vi "PulseParseCamera.vi"(0 "Pars String":string) -> (1 "aux camera pars":T1, 2 "main camera pars":T2)   [LabVIEW 2017]
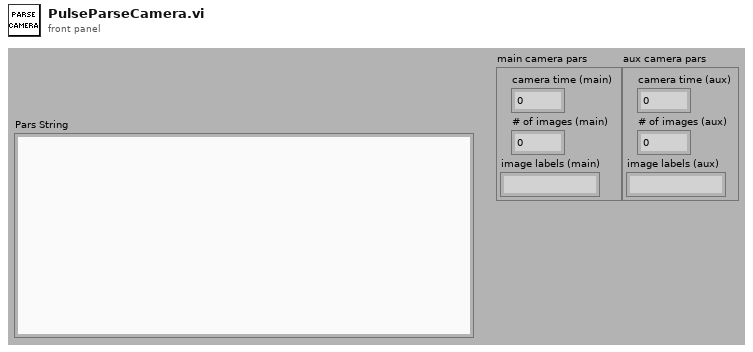
[diagram p1: front panel]
types:
  T1 = cluster{"camera time (aux)":i32, "# of images (aux)":i32, "image labels (aux)":string}
  T2 = cluster{"camera time (main)":i32, "# of images (main)":i32, "image labels (main)":string}
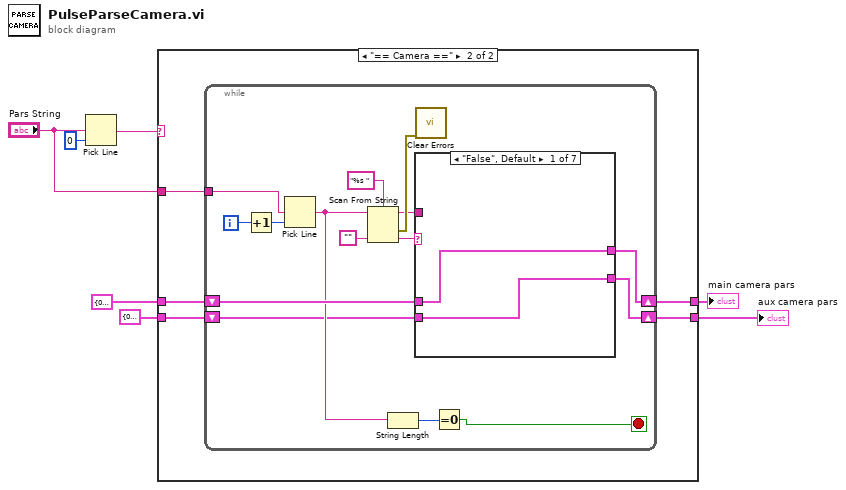
[diagram p0: block diagram]
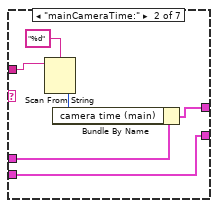
[diagram p3: hidden frame]
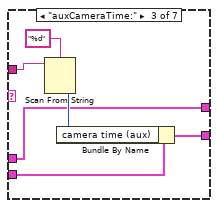
[diagram p4: hidden frame]
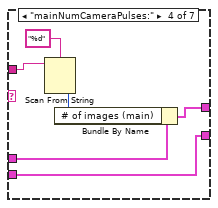
[diagram p5: hidden frame]
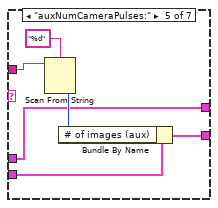
[diagram p6: hidden frame]
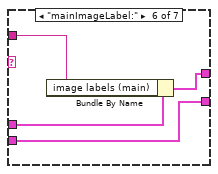
[diagram p7: hidden frame]
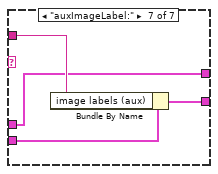
[diagram p8: hidden frame]
diagram:
  n1 = Pick Line(multi-line string="Pars String", line index=0) -> (output string=w6:string)  [unwired: 1 in]
  n2 = case shown="\"== Camera ==\"" w6 {
    tunnel: T2 {"camera time (main)"=0, "# of images (main)"=0, "image labels (main)"=""} ("Pars cluster 2") -> [w9 w14]
    tunnel: [w9 w13] -> w2
    tunnel: "Pars String" -> [_ w12]
    tunnel: T1 {"camera time (aux)"=0, "# of images (aux)"=0, "image labels (aux)"=""} ("Pars cluster 2") -> [w8 w11]
    tunnel: [w8 w10] -> w1
    frame "False", Default {
    }
    frame "== Camera ==" {
      n3 = while {
        shift-right: [w23] -> w13
        shift-left: w14 -> [w24]
        tunnel: w12 -> [w22]
        shift-right: [w15] -> w10
        shift-left: w11 -> [w16]
        i -> [w28]
        stop <- w19 stop-if-true
        n4 = Increment(x=w28) -> (x+1=w29:i32)
        n5 = Pick Line(multi-line string=w22, line index=w29) -> (output string=w21:string)  [unwired: 1 in]
        n6 = Scan From String(format string="%s ", input string=w21, default 1="") -> (remaining string=w17:string, error out=w18:errorcluster, output 1=w25:string)  [unwired: 2 in, 1 out]
        n7 = String Length(string=w21) -> (length=w20:i32)
        n8 = case shown="\"False\", Default" w25 {
          tunnel: w24 -> [w31 w36 w38 w48 w50 w59 w60]
          tunnel: [w31 w37 w38 w49 w50 w58 w60] -> w23
          tunnel: w17 -> [_ w34 w42 w46 w54 w57 w63]
          tunnel: w16 -> [w30 w32 w40 w44 w52 w56 w62]
          tunnel: [w30 w32 w39 w44 w51 w56 w61] -> w15
          frame "False", Default {
          }
          frame "mainCameraTime:" {
            n9 = Scan From String(format string="%d", input string=w34) -> (output 1=w33:i32)  [unwired: 3 in, 3 out]
            n10 = Bundle By Name(cluster=w36, "camera time (main)"=w33) -> (w37:T2)
          }
          frame "auxCameraTime:" {
            n11 = Scan From String(format string="%d", input string=w42) -> (output 1=w41:i32)  [unwired: 3 in, 3 out]
            n12 = Bundle By Name(cluster=w40, "camera time (aux)"=w41) -> (w39:T1)
          }
          frame "mainNumCameraPulses:" {
            n13 = Scan From String(format string="%d", input string=w46) -> (output 1=w45:i32)  [unwired: 3 in, 3 out]
            n14 = Bundle By Name(cluster=w48, "# of images (main)"=w45) -> (w49:T2)
          }
          frame "auxNumCameraPulses:" {
            n15 = Scan From String(format string="%d", input string=w54) -> (output 1=w53:i32)  [unwired: 3 in, 3 out]
            n16 = Bundle By Name(cluster=w52, "# of images (aux)"=w53) -> (w51:T1)
          }
          frame "mainImageLabel:" {
            n17 = Bundle By Name(cluster=w59, "image labels (main)"=w57) -> (w58:T2)
          }
          frame "auxImageLabel:" {
            n18 = Bundle By Name(cluster=w62, "image labels (aux)"=w63) -> (w61:T1)
          }
        }
        n19 = call <vilib>:"Clear Errors.vi"("error in (no error)"=w18) -> ()  [unwired: 5 in, 2 out]
        n20 = Equal To 0?(x=w20) -> (x = 0?=w19:bool)
      }
    }
  }
  "main camera pars" <- w2
  "aux camera pars" <- w1
